vi "Create Project.vi"(4 "error in":errorcluster, 6 "Project Definition":T1, 7 "Path":path) -> (0 "error out":errorcluster)   [LabVIEW 2025]
doc: "This VI creates a project according to the provided <b>Project Definition</b>, setting the project name, the description and all elements."
uses:
  Project Definition--cluster.ctl
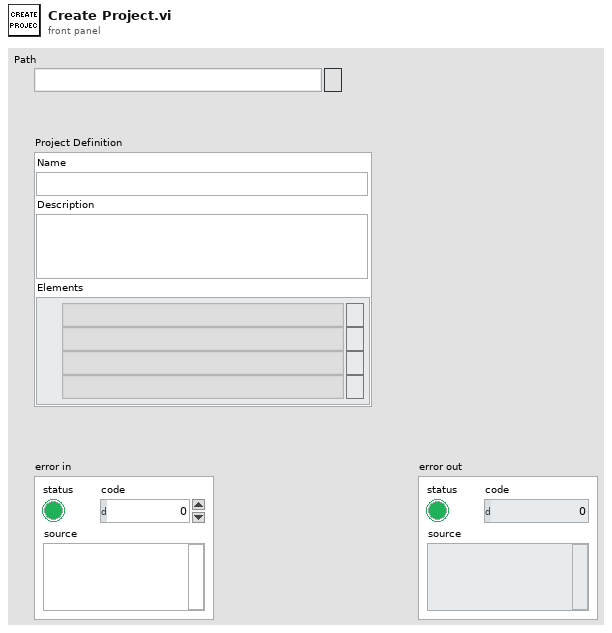
[diagram p1: front panel]
types:
  T1 = typedef "Project Definition--cluster.ctl" = cluster{"Name":string, "Description":string, "Elements":path[]}
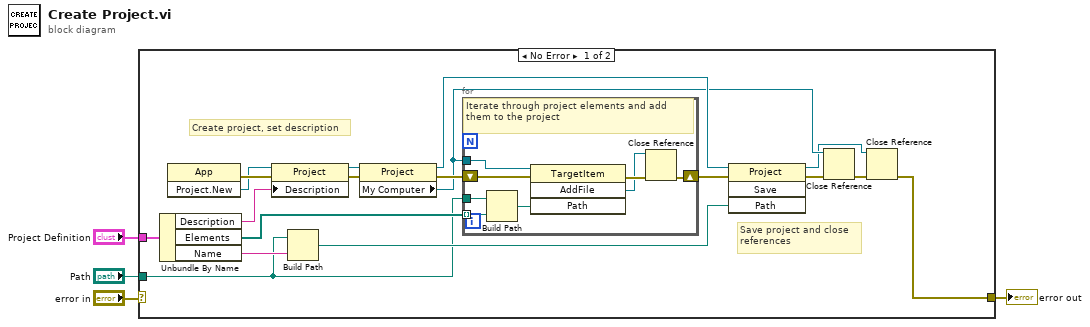
[diagram p0: block diagram]
diagram:
  n1 = case shown="No Error" "error in" {
    selector: "error in" -> [_ w31]
    tunnel: "Project Definition" -> [w13 _]
    tunnel: [w16 w31] -> w3
    tunnel: "Path" -> [w5 _]
    frame No Error {
      # "Save project and close \nreferences"
      # "Create project, set description"
      n2 = Unbundle By Name(w13) -> ("Description"=w7:string, "Elements"=w6:path[], "Name"=w9:string)
      n3 = invoke class="App" method="Project.New"() -> (error out=w22:errorcluster, "Project:New"=w15:refnum<vi>)  [unwired: 3 in, 1 out]
      n4 = property class="Project"(reference=w15, error in=w22, "Description"=w7) -> (reference out=w14:refnum<vi>, error out=w21:errorcluster)
      n5 = Build Path(base path=w5, name or relative path=w9) -> (appended path=w8:path)
      n6 = property class="Project"(reference=w14, error in=w21) -> (reference out=w12:refnum<vi>, error out=w20:errorcluster, "My Computer"=w11:refnum<vi>)
      n7 = for {
        tunnel: w11 -> [w27]
        shift-right: [w28] -> w19
        shift-left: w20 -> [w30]
        tunnel: w6 -> [w24] mode=indexing
        tunnel: w5 -> [w25]
        # "Iterate through project elements and add  them to the project"
        n8 = Build Path(base path=w25, name or relative path=w24) -> (appended path=w23:path)
        n9 = invoke class="TargetItem" method="AddFile"(reference=w27, error in=w30, "Path"=w23) -> (error out=w29:errorcluster, "AddFile"=w26:refnum<vi>)  [unwired: 1 in, 2 out]
        n10 = Close Reference(reference=w26, error in (no error)=w29) -> (error out=w28:errorcluster)
      }
      n11 = invoke class="Project" method="Save"(reference=w12, error in=w19, "Path"=w8) -> (reference out=w10:refnum<vi>, error out=w18:errorcluster)  [unwired: 1 in, 2 out]
      n12 = Close Reference(reference=w11, error in (no error)=w18) -> (error out=w17:errorcluster)
      n13 = Close Reference(reference=w10, error in (no error)=w17) -> (error out=w16:errorcluster)
    }
    frame Error {
      # "Pass error without further action"
    }
  }
  "error out" <- w3
